vi "Word_Insert_Control.vi"(0 "Word.Document":refnum<k7>, 1 "Word.InlineShapes":refnum<k7>, 2 "image depth":T2=3 items=["B&W", "4 bits", "8 bits", "24 bits"], 5 "Ctl Refnum":refnum<vi>, 7 "image file type(.jpg)":enum16{".jpg", ".png"}(ring), 9 "alignment (default)":T1, 11 "error in":errorcluster, 12 "Insertion point":u16(ring)=1 items=["begining of document", "end of document", "bookmark", "Custom"], 13 "bookmark name":string) -> (8 "Start out":i32, 10 "End out":i32, 15 "error out":errorcluster)   [LabVIEW 2010, in "NI_ReportGenerationToolkit.lvlib"]
uses:
  <vilib>/addons/_office/NI_ReportGenerationToolkit.lvlib
  <vilib>/Utility/NIReport.llb/image depth.ctl
  <vilib>/Utility/NIReport.llb/HTML Report Image Alignment.ctl
  <vilib>/Utility/NIReport.llb/NI_ReportGenerationCore.lvlib
panel:
  in  "Background color":u32(colorbox)=16777215
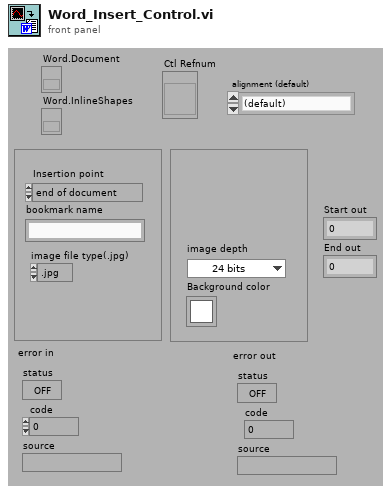
[diagram p1: front panel]
types:
  T1 = typedef "NI_ReportGenerationCore.lvlib/HTML Report Image Alignment.ctl" = enum16{"(default)", "LEFT", "RIGHT", "TOP", "TEXTTOP", "MIDDLE", "ABSMIDDLE", "BASELINE", "BOTTOM", "ABSBOTTOM"}
  T2 = typedef "NI_ReportGenerationCore.lvlib/image depth.ctl" = u16
  T3 = typedef "imagedata.ctl" = cluster{"image type":i32, "image depth":i32, "image":u8[], "mask":u8[], "colors":u32[], "Rectangle":cluster{"left":i16, "top":i16, "right":i16, "bottom":i16}}
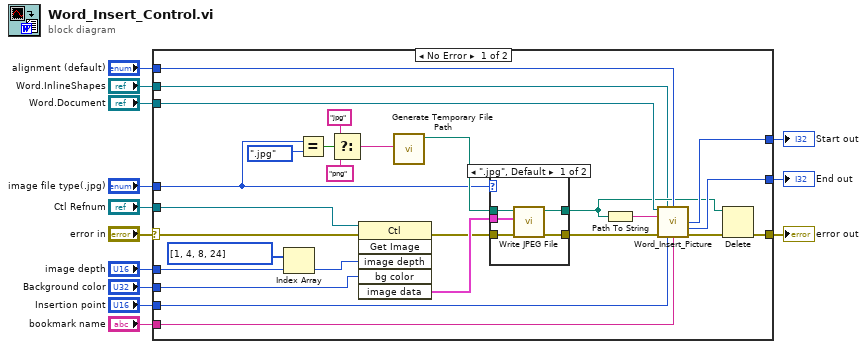
[diagram p0: block diagram]
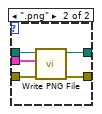
[diagram p2: hidden frame]
diagram:
  n1 = case shown="No Error" "error in" {
    selector: "error in" -> [w24 w51]
    tunnel: "image depth" -> [w39 _]
    tunnel: "Background color" -> [w37 _]
    tunnel: "Insertion point" -> [w34 _]
    tunnel: [w33 w51] -> w10
    tunnel: "bookmark name" -> [w32 _]
    tunnel: [w30 _] -> w8
    tunnel: [w29 _] -> w7
    tunnel: "Word.Document" -> [w28 _]
    tunnel: "Ctl Refnum" -> [w27 _]
    tunnel: "Word.InlineShapes" -> [w21 _]
    tunnel: "image file type(.jpg)" -> [w14 _]
    tunnel: "alignment (default)" -> [w26 _]
    frame No Error {
      n2 = Index Array(array=i32[] [1, 4, 8, 24] ("Array Constant"), index=w39) -> (element=w38:i32)
      n3 = Equal?(x=w14, y=enum16{".jpg", ".png"}.".jpg") -> (x = y?=w19:bool)
      n4 = Select(t="jpg", s=w19, f="png") -> (s? t:f=w18:string)
      n5 = invoke class="Ctl" method="Get Image"(reference=w27, error in=w24, "image depth"=w38, "bg color"=w37) -> (error out=w25:errorcluster, "image data"=w36:T3)  [unwired: 2 in, 4 out]
      n6 = call <vilib>:"Generate Temporary File Path.vi"("Temporary File Extension (tmp)"=w18) -> ("Unique Temporary File Path"=w15:path)  [unwired: 1 in, 9 out]
      n7 = case shown="\".jpg\", Default" w14 {
        tunnel: w36 -> [w41 w46]
        tunnel: w25 -> [w43 w50]
        tunnel: [w45 w49] -> w35
        tunnel: [w44 w48] -> w22
        tunnel: w15 -> [w42 w47]
        frame ".jpg", Default {
          n8 = call <vilib>:"Write JPEG File.vi"("error in (no error)"=w43, "image data"=w41, "path to JPEG file"=w42) -> ("error out"=w45:errorcluster, "path"=w44:path)  [unwired: 7 out]
        }
        frame ".png" {
          n9 = call <vilib>:"Write PNG File.vi"("error in (no error)"=w50, "image data"=w46, "path to PNG file"=w47) -> ("error out"=w49:errorcluster, "path"=w48:path)  [unwired: 1 in, 6 out]
        }
      }
      n10 = Path To String(path=w22) -> (string=w23:string)
      n11 = call <vilib>:"Word_Insert_Picture.vi"("Word.Document"=w28, "Word.InlineShapes"=w21, "alignment (default)"=w26, "Image file path"=w23, "error in (no error)"=w35, "Insertion point"=w34, "bookmark name"=w32) -> ("Start out"=w30:i32, "End out"=w29:i32, "error out 2"=w31:errorcluster)  [unwired: 2 in, 4 out]
      n12 = Delete(path (use dialog)=w22, error in=w31) -> (error out=w33:errorcluster)  [unwired: 5 out]
    }
    frame Error {
    }
  }
  "error out" <- w10
  "Start out" <- w8
  "End out" <- w7
